vi "GT Set Pid.vi"(7 "pPid":T1, 8 "error in (no error)":errorcluster caption="错误输入（无错误）", 9 "index":i16, 10 "control":i16, 11 "cardNum":i16) -> (0 "error out":errorcluster caption="错误输出", 3 "function return":i16, 5 "pPid out":T1)   [LabVIEW 2014, in "gts.lvlib"]
doc: "GT_API GT_SetPid(short cardNum,short control,short index,TPid *pPid);"
uses:
  gts.lvlib
  gts.dll
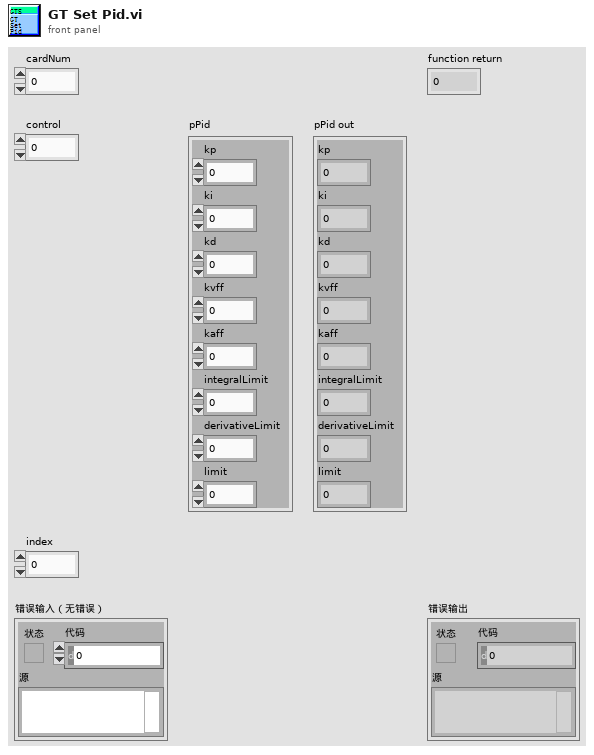
[diagram p1: front panel]
types:
  T1 = cluster{"kp":dbl, "ki":dbl, "kd":dbl, "kvff":dbl, "kaff":dbl, "integralLimit":i32, "derivativeLimit":i32, "limit":i16}
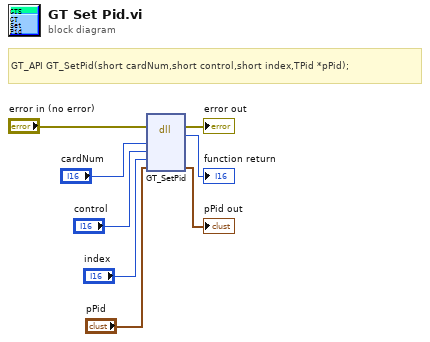
[diagram p0: block diagram]
diagram:
  # "GT_API GT_SetPid(short cardNum,short control,short index,TPid *pPid);"
  n1 = dll-call lib="PTH2?abs D\t王淼清$控制卡常用功能例程(Labview)gts.*" fn="GT_SetPid"(error in="error in (no error)", "cardNum"="cardNum", "control"="control", "index"="index", "pPid"="pPid") -> (error out=→"error out":errorcluster, →"function return":i16, "pPid"=→"pPid out":T1)  [unwired: 5 in, 1 out]
